vi "Proceed.vi"(7 "component is ready (Y)":bool=TRUE, 8 "error in (no error)":errorcluster, 10 "ProceedMessage":refnum<class "ProceedMessage.lvclass">, 11 "RSA in":refnum<class "RSA.lvclass">) -> (0 "error out":errorcluster, 2 "all observers are ready?":bool, 3 "RSA out":refnum<class "RSA.lvclass">)   [LabVIEW 2012, in "RSA.lvclass"]
uses:
  RSA.lvclass
  <vilib>/Distrio/Murmex/ProceedMessage/ProceedMessage.lvclass
  RSA.lvclass/RSA.ctl
  <vilib>/Distrio/Murmex/Murmex/Murmex.lvclass
  <vilib>/Analysis/NI_AALBase.lvlib
panel:
  # "This method is called when the PROCEED\ntrigger is sent. \n\nOverride this method when your component needs to\nrespond to this trigger. \n\nCall parent for proper implementation"
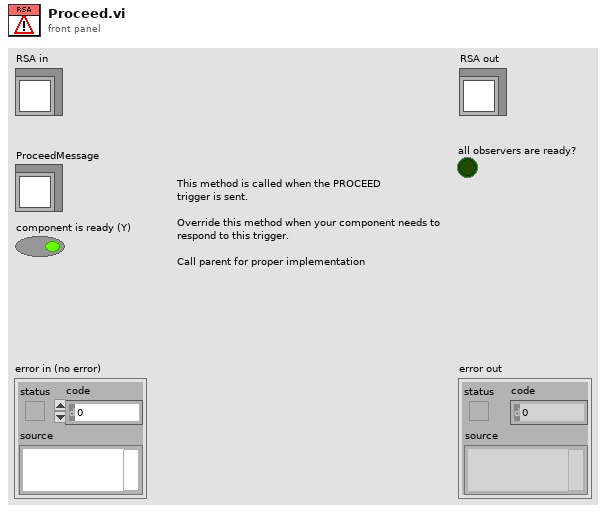
[diagram p1: front panel]
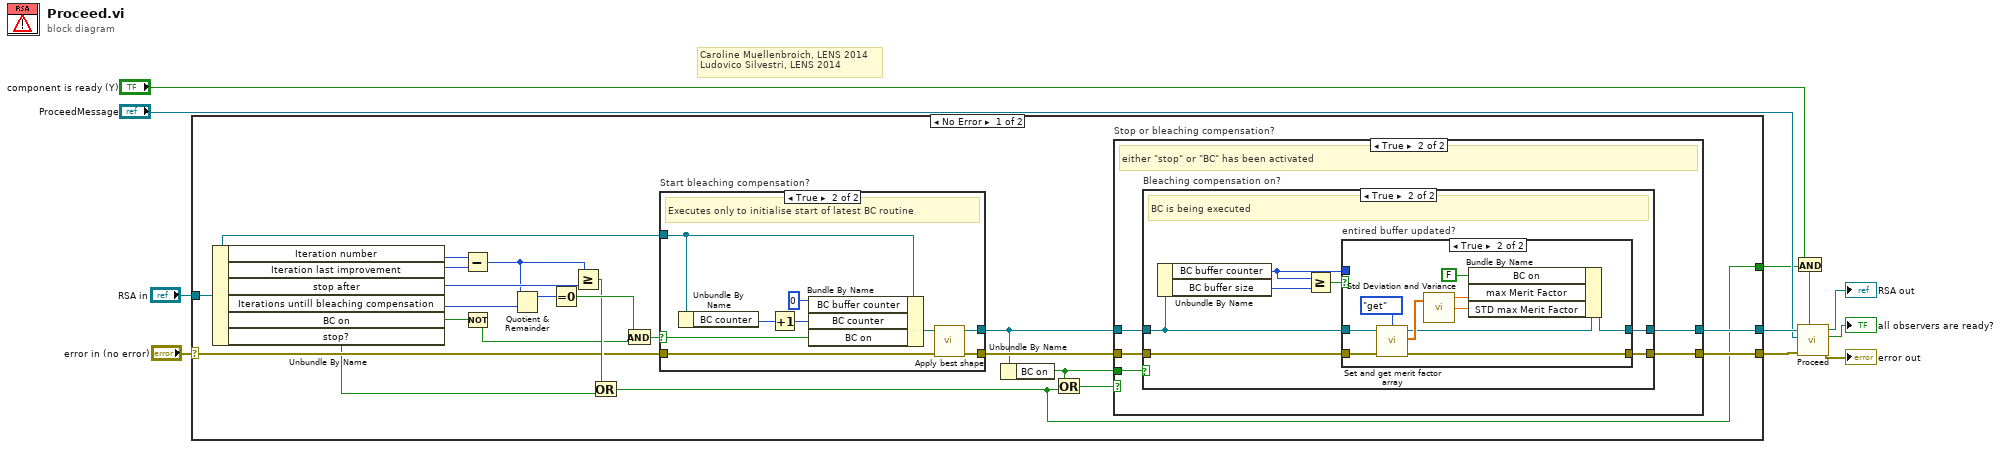
[diagram p0: block diagram]
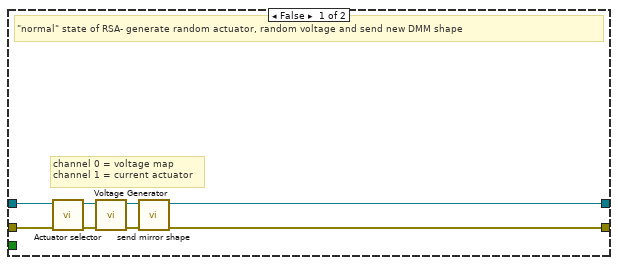
[diagram p3: hidden frame]
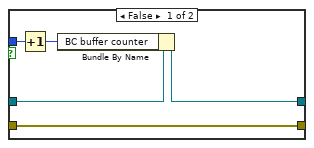
[diagram p5: hidden frame]
diagram:
  # "Caroline Muellenbroich, LENS 2014\nLudovico Silvestri, LENS 2014"
  n1 = case shown="No Error" "error in (no error)" {
    selector: "error in (no error)" -> [w25 w82]
    tunnel: [w23 w82] -> w7
    tunnel: "RSA in" -> [w14 w81]
    tunnel: [w24 w81] -> w5
    tunnel: [w12 _] -> w1
    frame No Error {
      n2 = Unbundle By Name(w14) -> ("Iteration number"=w13:i32, "Iteration last improvement"=w19:i32, "stop after"=w32:i32, "Iterations untill bleaching compensation"=w29:i32, "BC on"=w17:bool, "stop?"=w18:bool)
      n3 = Subtract(x=w13, y=w19) -> (x-y=w30:i32)
      n4 = Not(x=w17) -> (.not. x?=w15:bool)
      n5 = Quotient & Remainder(x=w30, y=w29) -> (x-y*floor(x/y)=w28:i32)  [unwired: 1 out]
      n6 = Equal To 0?(x=w28) -> (x = 0?=w27:bool)
      n7 = Greater Or Equal?(x=w30, y=w32) -> (x >= y?=w26:bool)
      n8 = Or(x=w26, y=w18) -> (x .or. y?=w12:bool)
      n9 = And(x=w27, y=w15) -> (x .and. y?=w16:bool)
      n10 = case "Start bleaching compensation?" shown="True" w16 {
        selector: w16 -> [_ w43]
        tunnel: w14 -> [w33 w42]
        tunnel: [w33 w36] -> w22
        tunnel: w25 -> [w34 w39]
        tunnel: [w34 w38] -> w31
        frame False {
        }
        frame True {
          # "Executes only to initialise start of latest BC routine"
          n11 = Unbundle By Name(w42) -> ("BC counter"=w41:i32)
          n12 = Increment(x=w41) -> (x+1=w40:i32)
          n13 = Bundle By Name(cluster=w42, "BC buffer counter"=0 ("Run time cluster.BC buffer counter"), "BC counter"=w40, "BC on"=w43) -> (w37:refnum<class "RSA.lvclass">)
          n14 = call "Apply best shape.vi"("error in (no error)"=w39, "RSA in"=w37) -> ("error out"=w38:errorcluster, "RSA out"=w36:refnum<class "RSA.lvclass">)  [unwired: 8 in]
        }
      }
      n15 = Unbundle By Name(w22) -> ("BC on"=w20:bool)
      n16 = Or(x=w20, y=w12) -> (x .or. y?=w21:bool)
      n17 = case "Stop or bleaching compensation?" shown="True" w21 {
        tunnel: w31 -> [w47 w54]
        tunnel: w22 -> [w44 w52]
        tunnel: [w46 w53] -> w24
        tunnel: [w45 w55] -> w23
        tunnel: w20 -> [_ w56]
        frame False {
          # "channel 0 = voltage map\nchannel 1 = current actuator"
          # "\"normal\" state of RSA- generate random actuator, random voltage and send new DMM shape"
          n18 = call-dynamic "Actuator selector.vi"("error in (no error)"=w47, "RSA in"=w44) -> ("error out"=w50:errorcluster, "RSA out"=w51:refnum<class "RSA.lvclass">)  [unwired: 8 in]
          n19 = call "Voltage Generator.vi"("error in (no error)"=w50, "RSA in"=w51) -> ("error out"=w49:errorcluster, "RSA out"=w48:refnum<class "RSA.lvclass">)  [unwired: 8 in]
          n20 = call-dynamic "send mirror shape.vi"("error in (no error)"=w49, "RSA in"=w48) -> ("error out"=w45:errorcluster, "RSA out"=w46:refnum<class "RSA.lvclass">)  [unwired: 8 in]
        }
        frame True {
          # "either \"stop\" or \"BC\" has been activated"
          n21 = case "Bleaching compensation on?" shown="True" w56 {
            tunnel: [w58 w61] -> w55
            tunnel: w54 -> [w58 w63]
            tunnel: [w57 w60] -> w53
            tunnel: w52 -> [w57 w62]
            frame False {
              # "Stop is being executed- do nothgin"
            }
            frame True {
              # "BC is being executed"
              n22 = Unbundle By Name(w62) -> ("BC buffer counter"=w59:i32, "BC buffer size"=w65:i32)
              n23 = Greater Or Equal?(x=w59, y=w65) -> (x >= y?=w64:bool)
              n24 = case "entired buffer updated?" shown="True" w64 {
                tunnel: w63 -> [w68 w78]
                tunnel: w62 -> [w70 w77]
                tunnel: [w68 w73] -> w61
                tunnel: [w69 w71] -> w60
                tunnel: w59 -> [w67 _]
                frame False {
                  n25 = Increment(x=w67) -> (x+1=w66:i32)
                  n26 = Bundle By Name(cluster=w70, "BC buffer counter"=w66) -> (w69:refnum<class "RSA.lvclass">)
                }
                frame True {
                  n27 = call "Set and get merit factor array.vi"("action"=enum16{"set", "get", "initialise"}."get", "error in (no error)"=w78, "RSA in"=w77) -> ("error out"=w73:errorcluster, "merit factor array"=w80:dbl[], "RSA out"=w72:refnum<class "RSA.lvclass">)  [unwired: 5 in, 1 out]
                  n28 = call <vilib>:"Std Deviation and Variance.vi"("X"=w80) -> ("mean"=w74:dbl, "standard deviation"=w75:dbl)  [unwired: 1 in, 1 out]
                  n29 = Bundle By Name(cluster=w72, "BC on"=FALSE ("Run time cluster.BC on"), "max Merit Factor"=w74, "STD max Merit Factor"=w75) -> (w71:refnum<class "RSA.lvclass">)
                }
              }
            }
          }
        }
      }
    }
    frame Error {
    }
  }
  n30 = And(x="component is ready (Y)", y=w1) -> (x .and. y?=w2:bool)
  n31 = call-parent "Proceed.vi"("component is ready (Y)"=w2, "error in (no error)"=w7, "ProceedMessage"="ProceedMessage", "Murmex in"=w5) -> ("error out"=→"error out":errorcluster, "all observers are ready?"=→"all observers are ready?":bool, "Murmex out"=→"RSA out":refnum<class "RSA.lvclass">)  [unwired: 5 in]
